vi "popUPCrearNuevoObjetoProducto.vi"() -> (3 "Listo Ingresar objeto Producto":bool=TRUE)   [LabVIEW 2014]
panel:
  in  "idRecipe":string="numLote"
  in  "dateCreate":string="dateCreate"
  in  "idProducto":string="idProducto"
  in  "objetoProducto":T1
  in  "textoFinCarga":string="Creando el nuevo objeto producto"
  in  "ingresarLote":string="numLote"
  in  "ingresarSteelGrade":string="numSteelGrade"
  in  "ingresarOD":string="numeroOD"
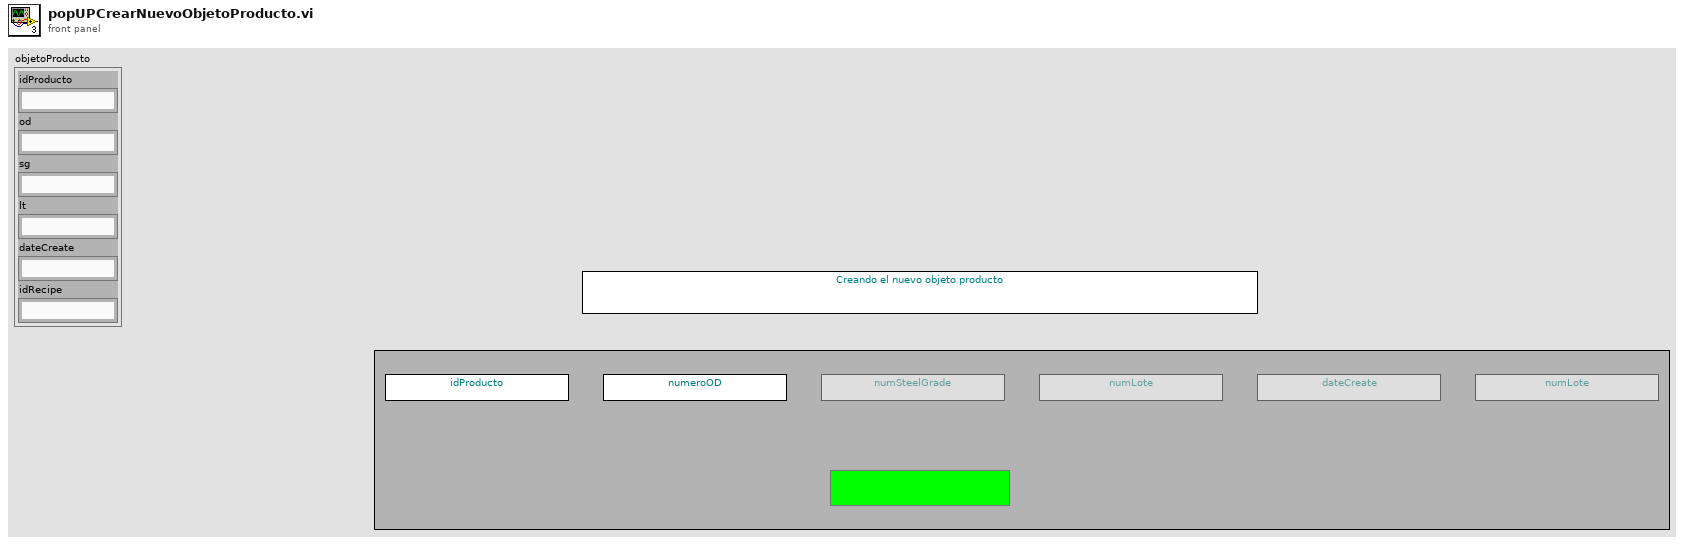
[diagram p1: front panel]
types:
  T1 = cluster{"idProducto":string, "od":string, "sg":string, "lt":string, "dateCreate":string, "idRecipe":string}
  T2 = enum8{"Enabled", "Disabled", "Disabled and Grayed Out"}
  T3 = cluster{"od":string, "sg":string, "lt":string, "idProducto":string, "dateCreate":string, "idRecipe":string}
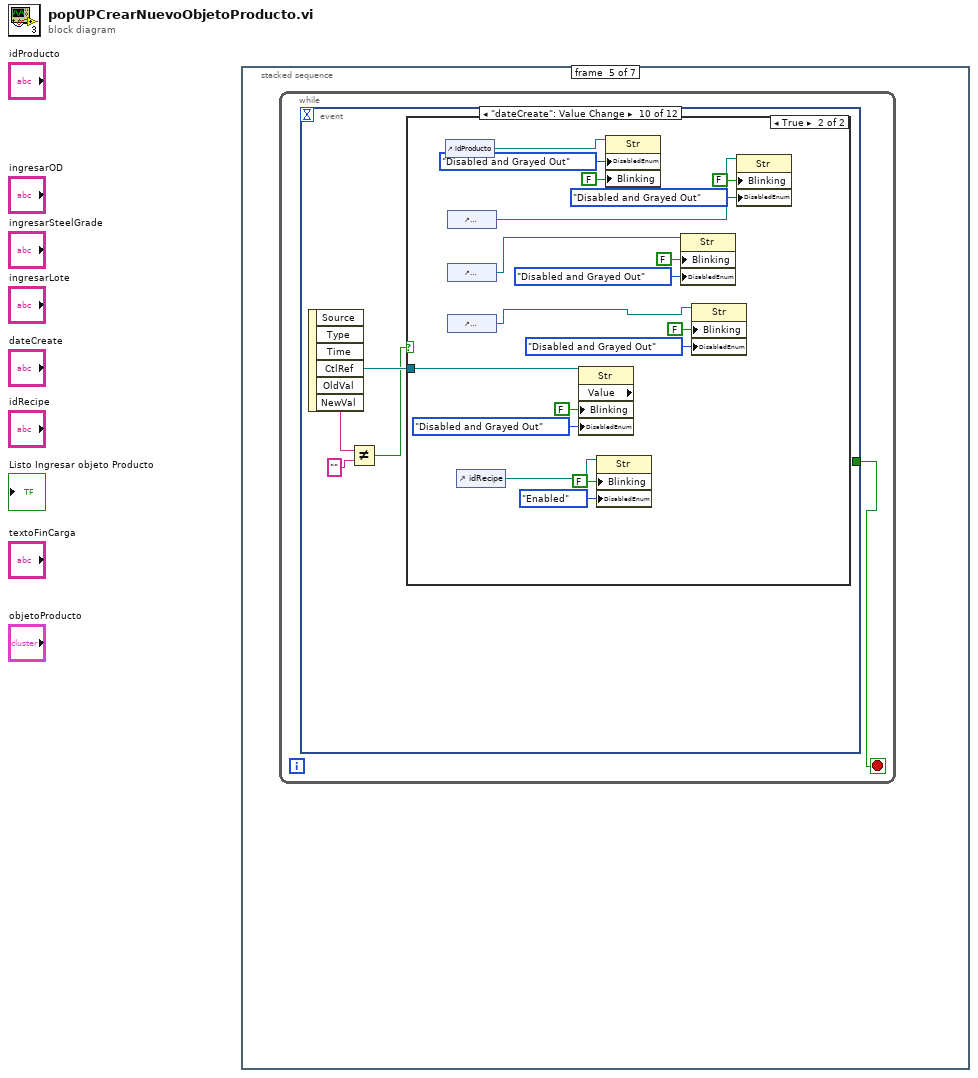
[diagram p0: block diagram]
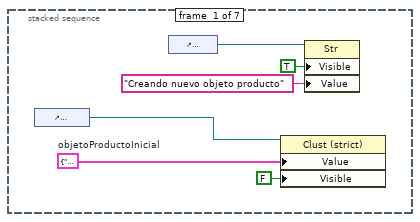
[diagram p2: hidden frame]
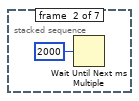
[diagram p3: hidden frame]
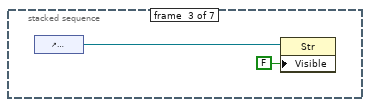
[diagram p4: hidden frame]
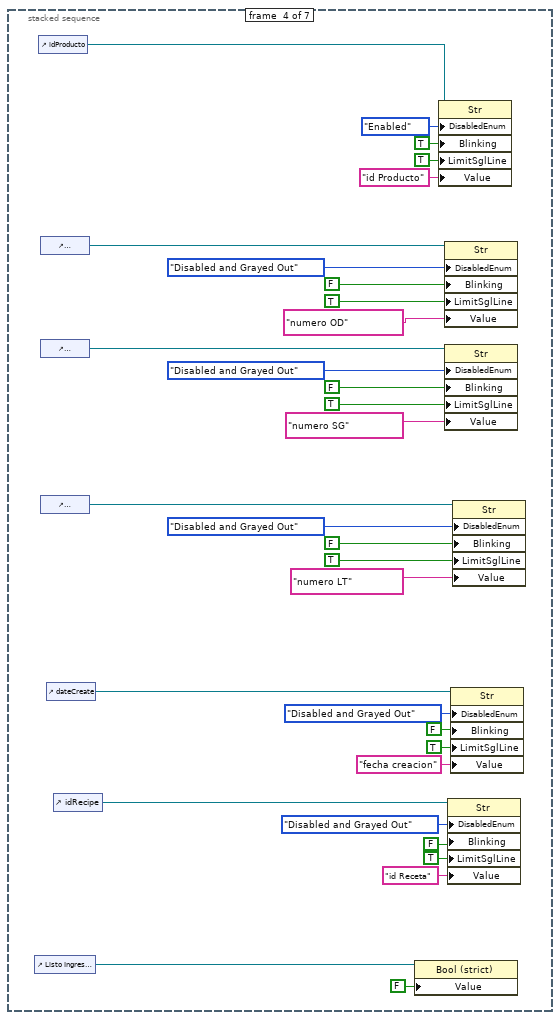
[diagram p5: hidden frame]
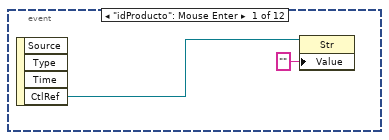
[diagram p6: hidden frame]
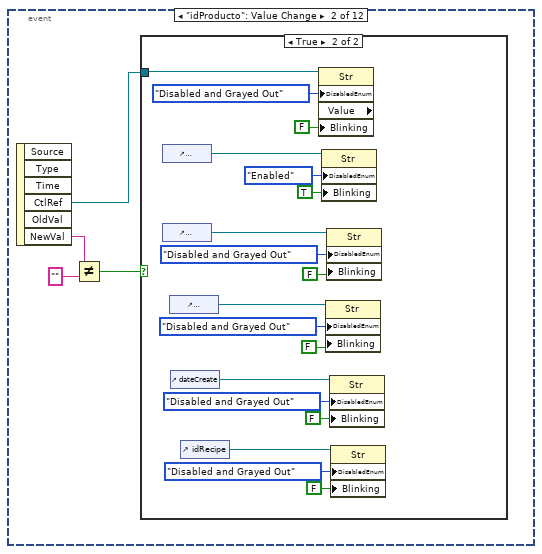
[diagram p7: hidden frame]
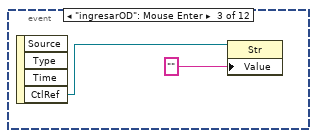
[diagram p9: hidden frame]
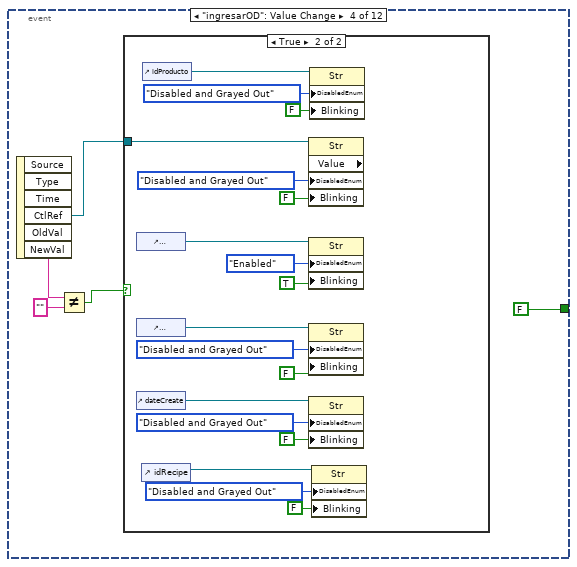
[diagram p10: hidden frame]
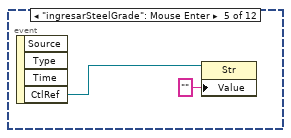
[diagram p12: hidden frame]
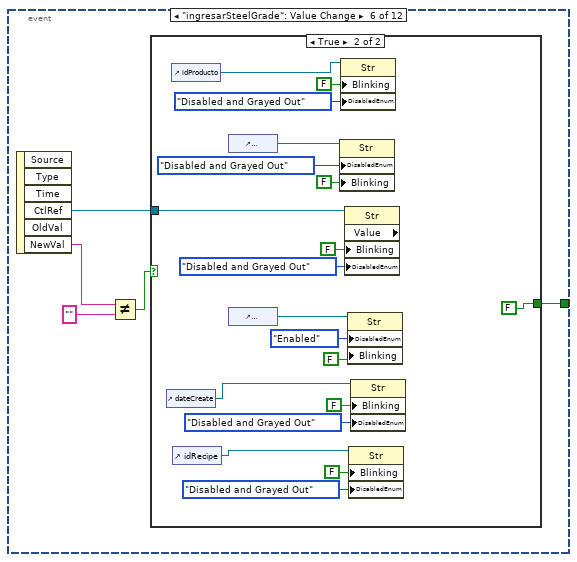
[diagram p13: hidden frame]
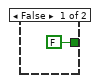
[diagram p14: hidden frame]
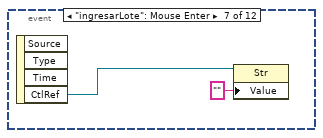
[diagram p15: hidden frame]
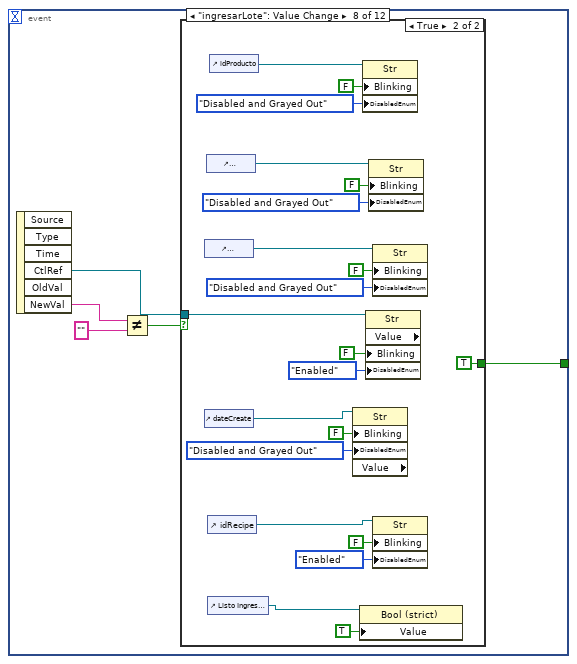
[diagram p16: hidden frame]
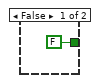
[diagram p17: hidden frame]
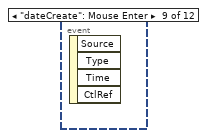
[diagram p18: hidden frame]
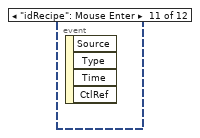
[diagram p20: hidden frame]
diagram:
  n1 = stacked-sequence {
    frame #0 {
      w1 = T1 {"idProducto"="", "od"="", "sg"="", "lt"="", "dateCreate"="", "idRecipe"=""}  # objetoProductoInicial
      n2 = control-ref of="objetoProducto"() -> (w2:refnum<vi>)
      n3 = control-ref of="textoFinCarga"() -> (w6:refnum<vi>)
      n4 = property class="Clust (strict)"(reference=w2, "Value"=w1, "Visible"=FALSE) -> ()  [unwired: 1 in, 2 out]
      n5 = property class="Str"(reference=w6, "Visible"=TRUE, "Value"="Creando nuevo objeto producto") -> ()  [unwired: 1 in, 2 out]
    }
    frame #1 {
      n6 = Wait Until Next ms Multiple(millisecond multiple=u32 2000) -> ()  [unwired: 1 out]
    }
    frame #2 {
      n7 = control-ref of="textoFinCarga"() -> (w9:refnum<vi>)
      n8 = property class="Str"(reference=w9, "Visible"=FALSE) -> ()  [unwired: 1 in, 2 out]
    }
    frame #3 {
      n9 = control-ref of="Listo Ingresar objeto Producto"() -> (w29:refnum<vi>)
      n10 = control-ref of="idProducto"() -> (w24:refnum<vi>)
      n11 = control-ref of="ingresarOD"() -> (w41:refnum<vi>)
      n12 = control-ref of="ingresarSteelGrade"() -> (w39:refnum<vi>)
      n13 = control-ref of="ingresarLote"() -> (w37:refnum<vi>)
      n14 = control-ref of="dateCreate"() -> (w19:refnum<vi>)
      n15 = control-ref of="idRecipe"() -> (w14:refnum<vi>)
      n16 = property class="Bool (strict)"(reference=w29, "Value"=FALSE) -> ()  [unwired: 1 in, 2 out]
      n17 = property class="Str"(reference=w24, "DisabledEnum"=T2."Enabled" ("Disabled"), "Blinking"=TRUE, "LimitSglLine"=TRUE ("Limit To Single Line?"), "Value"="id Producto") -> ()  [unwired: 1 in, 2 out]
      n18 = property class="Str"(reference=w41, "DisabledEnum"=T2."Disabled and Grayed Out" ("Disabled"), "Blinking"=FALSE, "LimitSglLine"=TRUE ("Limit To Single Line?"), "Value"="numero OD") -> ()  [unwired: 1 in, 2 out]
      n19 = property class="Str"(reference=w39, "DisabledEnum"=T2."Disabled and Grayed Out" ("Disabled"), "Blinking"=FALSE, "LimitSglLine"=TRUE ("Limit To Single Line?"), "Value"="numero SG") -> ()  [unwired: 1 in, 2 out]
      n20 = property class="Str"(reference=w14, "DisabledEnum"=T2."Disabled and Grayed Out" ("Disabled"), "Blinking"=FALSE, "LimitSglLine"=TRUE ("Limit To Single Line?"), "Value"="id Receta") -> ()  [unwired: 1 in, 2 out]
      n21 = property class="Str"(reference=w19, "DisabledEnum"=T2."Disabled and Grayed Out" ("Disabled"), "Blinking"=FALSE, "LimitSglLine"=TRUE ("Limit To Single Line?"), "Value"="fecha creacion") -> ()  [unwired: 1 in, 2 out]
      n22 = property class="Str"(reference=w37, "DisabledEnum"=T2."Disabled and Grayed Out" ("Disabled"), "Blinking"=FALSE, "LimitSglLine"=TRUE ("Limit To Single Line?"), "Value"="numero LT") -> ()  [unwired: 1 in, 2 out]
    }
    frame #4 {
      n23 = while {
        stop <- w42 stop-if-true
        n24 = event shown="[9] \"dateCreate\": Value Change" {
          selector: _ -> [_ _ _ _ _ _ _ _ _ _ _ _]
          dyn-events: _ -> [_ _ _ _ _ _ _ _ _ _ _ _]
          timeout: _ -> [_ _ _ _ _ _ _ _ _ _ _ _]
          tunnel: [_ _ _ FALSE _ w97 _ w124 _ _ _ _] -> w42
          event "idProducto": Mouse Enter {
            n25 = event-data() -> ("CtlRef"=w44:refnum<vi>)  [unwired: 1 in, 3 out]
            n26 = property class="Str"(reference=w44, "Value"="") -> ()  [unwired: 1 in, 2 out]
          }
          event "idProducto": Value Change {
            n27 = event-data() -> ("CtlRef"=w45:refnum<vi>, "NewVal"=w48:string)  [unwired: 1 in, 4 out]
            n28 = Not Equal?(x=w48, y="") -> (x != y?=w46:bool)
            n29 = case shown="True" w46 {
              tunnel: w45 -> [_ w66]
              frame False {
              }
              frame True {
                n30 = control-ref of="ingresarOD"() -> (w64:refnum<vi>)
                n31 = control-ref of="ingresarSteelGrade"() -> (w60:refnum<vi>)
                n32 = control-ref of="ingresarLote"() -> (w57:refnum<vi>)
                n33 = control-ref of="dateCreate"() -> (w54:refnum<vi>)
                n34 = control-ref of="idRecipe"() -> (w51:refnum<vi>)
                n35 = property class="Str" props=["DisabledEnum", "Value", "Blinking"](reference=w66, "DisabledEnum"=T2."Disabled and Grayed Out" ("Disabled"), "Blinking"=FALSE) -> ()  [unwired: 1 in, 3 out]
                n36 = property class="Str"(reference=w64, "DisabledEnum"=T2."Enabled" ("Disabled"), "Blinking"=TRUE) -> ()  [unwired: 1 in, 2 out]
                n37 = property class="Str"(reference=w57, "DisabledEnum"=T2."Disabled and Grayed Out" ("Disabled"), "Blinking"=FALSE) -> ()  [unwired: 1 in, 2 out]
                n38 = property class="Str"(reference=w60, "DisabledEnum"=T2."Disabled and Grayed Out" ("Disabled"), "Blinking"=FALSE) -> ()  [unwired: 1 in, 2 out]
                n39 = property class="Str"(reference=w54, "DisabledEnum"=T2."Disabled and Grayed Out" ("Disabled"), "Blinking"=FALSE) -> ()  [unwired: 1 in, 2 out]
                n40 = property class="Str"(reference=w51, "DisabledEnum"=T2."Disabled and Grayed Out" ("Disabled"), "Blinking"=FALSE) -> ()  [unwired: 1 in, 2 out]
              }
            }
          }
          event "ingresarOD": Mouse Enter {
            n41 = event-data() -> ("CtlRef"=w68:refnum<vi>)  [unwired: 1 in, 3 out]
            n42 = property class="Str"(reference=w68, "Value"="") -> ()  [unwired: 1 in, 2 out]
          }
          event "ingresarOD": Value Change {
            n43 = event-data() -> ("CtlRef"=w73:refnum<vi>, "NewVal"=w70:string)  [unwired: 1 in, 4 out]
            n44 = Not Equal?(x=w70, y="") -> (x != y?=w71:bool)
            n45 = case shown="True" w71 {
              tunnel: w73 -> [_ w91]
              frame False {
              }
              frame True {
                n46 = control-ref of="ingresarSteelGrade"() -> (w88:refnum<vi>)
                n47 = control-ref of="ingresarLote"() -> (w85:refnum<vi>)
                n48 = control-ref of="dateCreate"() -> (w82:refnum<vi>)
                n49 = control-ref of="idRecipe"() -> (w76:refnum<vi>)
                n50 = control-ref of="idProducto"() -> (w79:refnum<vi>)
                n51 = property class="Str" props=["Value", "DisabledEnum", "Blinking"](reference=w91, "DisabledEnum"=T2."Disabled and Grayed Out" ("Disabled"), "Blinking"=FALSE) -> ()  [unwired: 1 in, 3 out]
                n52 = property class="Str"(reference=w88, "DisabledEnum"=T2."Enabled" ("Disabled"), "Blinking"=TRUE) -> ()  [unwired: 1 in, 2 out]
                n53 = property class="Str"(reference=w85, "DisabledEnum"=T2."Disabled and Grayed Out" ("Disabled"), "Blinking"=FALSE) -> ()  [unwired: 1 in, 2 out]
                n54 = property class="Str"(reference=w82, "DisabledEnum"=T2."Disabled and Grayed Out" ("Disabled"), "Blinking"=FALSE) -> ()  [unwired: 1 in, 2 out]
                n55 = property class="Str"(reference=w79, "DisabledEnum"=T2."Disabled and Grayed Out" ("Disabled"), "Blinking"=FALSE) -> ()  [unwired: 1 in, 2 out]
                n56 = property class="Str"(reference=w76, "DisabledEnum"=T2."Disabled and Grayed Out" ("Disabled"), "Blinking"=FALSE) -> ()  [unwired: 1 in, 2 out]
              }
            }
          }
          event "ingresarSteelGrade": Mouse Enter {
            n57 = event-data() -> ("CtlRef"=w93:refnum<vi>)  [unwired: 1 in, 3 out]
            n58 = property class="Str"(reference=w93, "Value"="") -> ()  [unwired: 1 in, 2 out]
          }
          event "ingresarSteelGrade": Value Change {
            n59 = event-data() -> ("CtlRef"=w98:refnum<vi>, "NewVal"=w96:string)  [unwired: 1 in, 4 out]
            n60 = Not Equal?(x=w96, y="") -> (x != y?=w94:bool)
            n61 = case shown="True" w94 {
              tunnel: w98 -> [_ w118]
              tunnel: [FALSE FALSE] -> w97
              frame False {
              }
              frame True {
                n62 = control-ref of="dateCreate"() -> (w105:refnum<vi>)
                n63 = control-ref of="idProducto"() -> (w108:refnum<vi>)
                n64 = control-ref of="idRecipe"() -> (w102:refnum<vi>)
                n65 = control-ref of="ingresarOD"() -> (w116:refnum<vi>)
                n66 = control-ref of="ingresarLote"() -> (w113:refnum<vi>)
                n67 = property class="Str"(reference=w116, "DisabledEnum"=T2."Disabled and Grayed Out" ("Disabled"), "Blinking"=FALSE) -> ()  [unwired: 1 in, 2 out]
                n68 = property class="Str"(reference=w108, "Blinking"=FALSE, "DisabledEnum"=T2."Disabled and Grayed Out" ("Disabled")) -> ()  [unwired: 1 in, 2 out]
                n69 = property class="Str" props=["Value", "Blinking", "DisabledEnum"](reference=w118, "Blinking"=FALSE, "DisabledEnum"=T2."Disabled and Grayed Out" ("Disabled")) -> ()  [unwired: 1 in, 3 out]
                n70 = property class="Str"(reference=w113, "DisabledEnum"=T2."Enabled" ("Disabled"), "Blinking"=FALSE) -> ()  [unwired: 1 in, 2 out]
                n71 = property class="Str"(reference=w102, "Blinking"=FALSE, "DisabledEnum"=T2."Disabled and Grayed Out" ("Disabled")) -> ()  [unwired: 1 in, 2 out]
                n72 = property class="Str"(reference=w105, "Blinking"=FALSE, "DisabledEnum"=T2."Disabled and Grayed Out" ("Disabled")) -> ()  [unwired: 1 in, 2 out]
              }
            }
          }
          event "ingresarLote": Mouse Enter {
            n73 = event-data() -> ("CtlRef"=w120:refnum<vi>)  [unwired: 1 in, 3 out]
            n74 = property class="Str"(reference=w120, "Value"="") -> ()  [unwired: 1 in, 2 out]
          }
          event "ingresarLote": Value Change {
            n75 = event-data() -> ("CtlRef"=w125:refnum<vi>, "NewVal"=w123:string)  [unwired: 1 in, 4 out]
            n76 = Not Equal?(x=w123, y="") -> (x != y?=w122:bool)
            n77 = case shown="True" w122 {
              tunnel: w125 -> [_ w147]
              tunnel: [FALSE TRUE] -> w124
              frame False {
              }
              frame True {
                n78 = control-ref of="ingresarSteelGrade"() -> (w140:refnum<vi>)
                n79 = control-ref of="dateCreate"() -> (w132:refnum<vi>)
                n80 = control-ref of="ingresarOD"() -> (w143:refnum<vi>)
                n81 = control-ref of="idRecipe"() -> (w129:refnum<vi>)
                n82 = control-ref of="Listo Ingresar objeto Producto"() -> (w137:refnum<vi>)
                n83 = control-ref of="idProducto"() -> (w135:refnum<vi>)
                n84 = property class="Str" props=["Blinking", "DisabledEnum", "Value"](reference=w132, "Blinking"=FALSE, "DisabledEnum"=T2."Disabled and Grayed Out" ("Disabled")) -> ()  [unwired: 1 in, 3 out]
                n85 = property class="Bool (strict)"(reference=w137, "Value"=TRUE) -> ()  [unwired: 1 in, 2 out]
                n86 = property class="Str"(reference=w135, "Blinking"=FALSE, "DisabledEnum"=T2."Disabled and Grayed Out" ("Disabled")) -> ()  [unwired: 1 in, 2 out]
                n87 = property class="Str" props=["Value", "Blinking", "DisabledEnum"](reference=w147, "Blinking"=FALSE, "DisabledEnum"=T2."Enabled" ("Disabled")) -> ()  [unwired: 1 in, 3 out]
                n88 = property class="Str"(reference=w143, "Blinking"=FALSE, "DisabledEnum"=T2."Disabled and Grayed Out" ("Disabled")) -> ()  [unwired: 1 in, 2 out]
                n89 = property class="Str"(reference=w140, "Blinking"=FALSE, "DisabledEnum"=T2."Disabled and Grayed Out" ("Disabled")) -> ()  [unwired: 1 in, 2 out]
                n90 = property class="Str"(reference=w129, "Blinking"=FALSE, "DisabledEnum"=T2."Enabled" ("Disabled")) -> ()  [unwired: 1 in, 2 out]
              }
            }
          }
          event "dateCreate": Mouse Enter {
            n91 = event-data() -> ()  [unwired: 1 in, 4 out]
          }
          event "dateCreate": Value Change {
            n92 = event-data() -> ("CtlRef"=w151:refnum<vi>, "NewVal"=w149:string)  [unwired: 1 in, 4 out]
            n93 = Not Equal?(x=w149, y="" ("NewVal")) -> (x != y?=w150:bool)
            n94 = case shown="True" w150 {
              tunnel: w151 -> [_ w169]
              frame False {
              }
              frame True {
                n95 = control-ref of="idProducto"() -> (w166:refnum<vi>)
                n96 = control-ref of="ingresarOD"() -> (w155:refnum<vi>)
                n97 = control-ref of="ingresarSteelGrade"() -> (w160:refnum<vi>)
                n98 = control-ref of="ingresarLote"() -> (w163:refnum<vi>)
                n99 = control-ref of="idRecipe"() -> (w165:refnum<vi>)
                n100 = property class="Str" props=["Value", "Blinking", "DisabledEnum"](reference=w169, "Blinking"=FALSE, "DisabledEnum"=T2."Disabled and Grayed Out" ("Disabled")) -> ()  [unwired: 1 in, 3 out]
                n101 = property class="Str"(reference=w165, "Blinking"=FALSE, "DisabledEnum"=T2."Enabled" ("Disabled")) -> ()  [unwired: 1 in, 2 out]
                n102 = property class="Str"(reference=w166, "DisabledEnum"=T2."Disabled and Grayed Out" ("Disabled"), "Blinking"=FALSE) -> ()  [unwired: 1 in, 2 out]
                n103 = property class="Str"(reference=w160, "Blinking"=FALSE, "DisabledEnum"=T2."Disabled and Grayed Out" ("Disabled")) -> ()  [unwired: 1 in, 2 out]
                n104 = property class="Str"(reference=w163, "Blinking"=FALSE, "DisabledEnum"=T2."Disabled and Grayed Out" ("Disabled")) -> ()  [unwired: 1 in, 2 out]
                n105 = property class="Str"(reference=w155, "Blinking"=FALSE, "DisabledEnum"=T2."Disabled and Grayed Out" ("Disabled")) -> ()  [unwired: 1 in, 2 out]
              }
            }
          }
          event "idRecipe": Mouse Enter {
            n106 = event-data() -> ()  [unwired: 1 in, 4 out]
          }
          event "idRecipe": Value Change {
            n107 = event-data() -> ()  [unwired: 1 in, 6 out]
          }
        }
      }
    }
    frame #5 {
      n108 = control-ref of="textoFinCarga"() -> (w172:refnum<vi>)
      n109 = property class="Str"(reference=w172, "Value"="Gracias por ingresar los datos del producto", "Visible"=TRUE) -> ()  [unwired: 1 in, 2 out]
    }
    frame #6 {
      w182 = T3 {"od"="", "sg"="", "lt"="", "idProducto"="", "dateCreate"="", "idRecipe"=""}  # objetoProducto
      n110 = control-ref of="ingresarOD"() -> (w187:refnum<vi>)
      n111 = control-ref of="ingresarSteelGrade"() -> (w186:refnum<vi>)
      n112 = control-ref of="ingresarLote"() -> (w185:refnum<vi>)
      n113 = control-ref of="idProducto"() -> (w178:refnum<vi>)
      n114 = control-ref of="idRecipe"() -> (w174:refnum<vi>)
      n115 = control-ref of="dateCreate"() -> (w176:refnum<vi>)
      n116 = property class="Str"(reference=w187) -> ("Value"=w181:string)  [unwired: 1 in, 2 out]
      n117 = property class="Str"(reference=w186) -> ("Value"=w180:string)  [unwired: 1 in, 2 out]
      n118 = property class="Str"(reference=w174) -> ("Value"=w173:string)  [unwired: 1 in, 2 out]
      n119 = property class="Str"(reference=w185) -> ("Value"=w179:string)  [unwired: 1 in, 2 out]
      n120 = property class="Str"(reference=w178) -> ("Value"=w177:string)  [unwired: 1 in, 2 out]
      n121 = property class="Str"(reference=w176) -> ("Value"=w175:string)  [unwired: 1 in, 2 out]
      n122 = Wait Until Next ms Multiple(millisecond multiple=u32 2000) -> ()  [unwired: 1 out]
      n123 = Bundle(cluster=w182, "od"=w181, "sg"=w180, "lt"=w179, "idProducto"=w177, "dateCreate"=w175, "idRecipe"=w173) -> (w184:T3)
      n124 = control-ref of="objetoProducto"() -> (w183:refnum<vi>)
      n125 = property class="Clust (strict)"(reference=w183, "Value"=w184) -> ()  [unwired: 1 in, 2 out]
    }
  }
